vi "TDMS Buffer Size.vi"(8 "error in (no error)":errorcluster, 9 "group name in":string, 10 "Channel Names Array":string[](array[string]), 11 "Refnum in":refnum<k34>) -> (0 "error out":errorcluster)   [LabVIEW 2014, in "File IO.lvlib"]
uses:
  File IO.lvlib
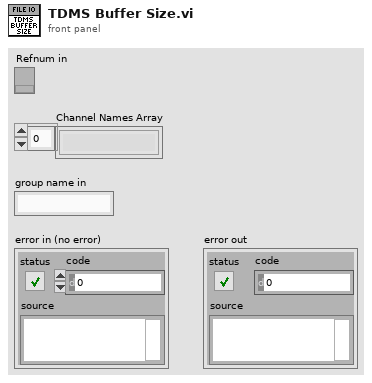
[diagram p1: front panel]
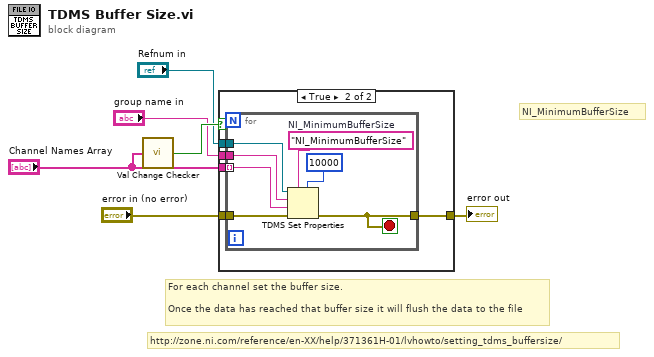
[diagram p0: block diagram]
diagram:
  # "http://zone.ni.com/reference/en-XX/help/371361H-01/lvhowto/setting_tdms_buffersize/"
  # "For each channel set the buffer size. \n\nOnce the data has reached that buffer size it will flush the data to the file"
  # "NI_MinimumBufferSize"
  n1 = call "Val Change Checker.vi"("Current Value in"="Channel Names Array") -> ("Value Change?"=w6:bool)
  n2 = case shown="True" w6 {
    tunnel: "Refnum in" -> [_ w12]
    tunnel: "group name in" -> [_ w11]
    tunnel: "error in (no error)" -> [w7 w10]
    tunnel: [w7 w9] -> w1
    tunnel: "Channel Names Array" -> [_ w8]
    frame False {
    }
    frame True {
      n3 = for {
        tunnel: w12 -> [w19]
        tunnel: w11 -> [w18]
        tunnel: w10 -> [w17]
        tunnel: [w13] -> w9
        tunnel: w8 -> [w16] mode=indexing
        stop <- w13 stop-if-true
        w15 = "NI_MinimumBufferSize"  # NI_MinimumBufferSize
        n4 = TDMS Set Properties(5:10000, 7:w15, 8:w17, 9:w16, 10:w18, 11:w19) -> (0:w13:errorcluster)  [unwired: 3 out]
      }
    }
  }
  "error out" <- w1
